vi "PSTR-Regenerate Best Fits.vi"(0 "PSTH":dbl[](array[numeric]), 5 "params":dbl[](array[numeric]), 7 "dt (ms)":dbl, 9 "delay (ms)":dbl, 11 "durat (ms)":dbl) -> (4 "t":dbl[](array[numeric]), 8 "y":dbl[](array[numeric]))   [LabVIEW 2020]
uses:
  epl-vi-lib/Utility VIs/Math VIs/LinSpace (x0-dx-npts).vi
  <vilib>/Analysis/baseanly.llb/Mean (DBL).vi
  <vilib>/Analysis/NI_AALBase.lvlib
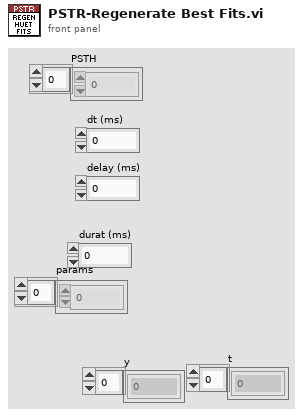
[diagram p1: front panel]
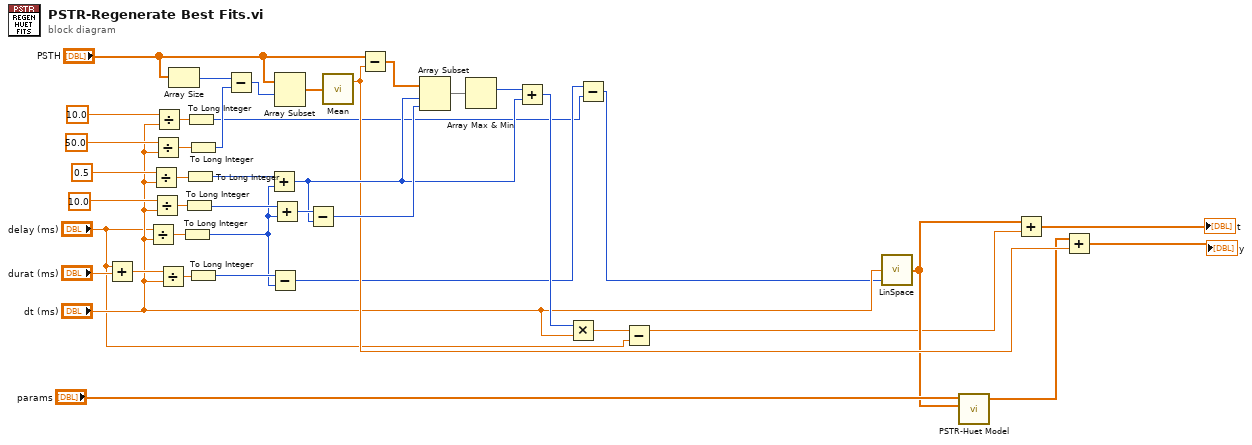
[diagram p0: block diagram]
diagram:
  n1 = Add(x="delay (ms)", y="durat (ms)") -> (x+y=w39:dbl)
  n2 = Divide(x="delay (ms)", y="dt (ms)") -> (x/y=w41:dbl)
  n3 = Divide(x=0.5, y="dt (ms)") -> (x/y=w35:dbl)
  n4 = Divide(x=10.0, y="dt (ms)") -> (x/y=w34:dbl)
  n5 = Divide(x=50.0, y="dt (ms)") -> (x/y=w25:dbl)
  n6 = Divide(x=10.0, y="dt (ms)") -> (x/y=w9:dbl)
  n7 = Divide(x=w39, y="dt (ms)") -> (x/y=w38:dbl)
  n8 = Array Size(array="PSTH") -> (size(s)=w23:i32)
  n9 = To Long Integer(number=w41) -> (32bit integer=w27:i32)
  n10 = To Long Integer(number=w34) -> (32bit integer=w33:i32)
  n11 = To Long Integer(number=w35) -> (32bit integer=w12:i32)
  n12 = To Long Integer(number=w9) -> (32bit integer=w8:i32)
  n13 = To Long Integer(number=w25) -> (32bit integer=w19:i32)
  n14 = To Long Integer(number=w38) -> (32bit integer=w28:i32)
  n15 = Subtract(x=w23, y=w19) -> (x-y=w20:i32)
  n16 = Add(x=w12, y=w27) -> (x+y=w18:i32)
  n17 = Subtract(x=w28, y=w27) -> (x-y=w13:i32)
  n18 = Add(x=w33, y=w27) -> (x+y=w29:i32)
  n19 = Array Subset(array="PSTH", index=w20) -> (w22:dbl[])  [unwired: 1 in]
  n20 = Subtract(x=w29, y=w18) -> (x-y=w32:i32)
  n21 = call-poly <vilib>:"Mean.vi"("X"=w22) -> ("mean"=w15:dbl)  [unwired: 1 out]
  n22 = Subtract(x="PSTH", y=w15) -> (x-y=w21:dbl[])
  n23 = Array Subset(array=w21, index=w18, length=w32) -> (w31:dbl[])
  n24 = Array Max & Min(array=w31) -> (max index (indices)=w30:i32)  [unwired: 3 out]
  n25 = Add(x=w30, y=w18) -> (x+y=w16:i32)
  n26 = Multiply(x=w16, y="dt (ms)") -> (x*y=w3:dbl)
  n27 = Subtract(x=w13, y=w8) -> (x-y=w7:i32)
  n28 = Subtract(x=w3, y="delay (ms)") -> (x-y=w2:dbl)
  n29 = call-poly "LinSpace.vi"("npts"=w7, "dx"="dt (ms)") -> ("Array"=w4:dbl[])  [unwired: 2 in, 1 out]
  n30 = call "PSTR-Huet Model.vi"("X"=w4, "a"="params") -> ("f(X,a)"=w5:dbl[])  [unwired: 2 in, 2 out]
  n31 = Add(x=w4, y=w2) -> (x+y=→"t":dbl[])
  n32 = Add(x=w5, y=w15) -> (x+y=→"y":dbl[])
